vi "CfgFile Create Language File Chinese.vi"(8 "error in (no error)":errorcluster, 11 "LF2R IDE in":refnum<class "LF2R IDE.lvclass">) -> (0 "error out":errorcluster, 3 "LF2R IDE out":refnum<class "LF2R IDE.lvclass">)   [LabVIEW 2018, in "LF2R IDE.lvlib" / "LF2R IDE.lvclass"]
uses:
  LF2R IDE.lvclass
  0fceaff6-5102-487b-a0d8-62e3909835e7.vi
  <vilib>/JDP Science/JSONtext/Variant to JSON Text.vi
  <vilib>/JDP Science/JSONtext/LVClass Serializer/JSONtext LVClass Serializer.lvclass
  <vilib>/JDP Science/JSONtext/JSONtext.lvlib
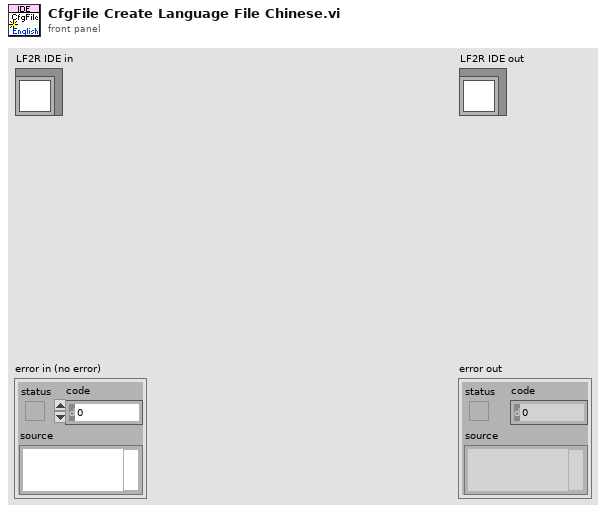
[diagram p1: front panel]
types:
  T1 = enum16{"open", "replace", "create", "open or create", "replace or create", "replace or create with confirmation"}
  T2 = typedef "LF2R IDE.lvlib/LF2R IDE.lvclass/Const UI Description Setting.ctl" = cluster{"Title":T3, "Frame Basic":T5, "Frame Skill":T6, "bp":T7, "w":T8, "b":T9, "i":T10, "o":T11, "c":T12, "Other":T13, "Menu":T14}
  T3 = typedef "LF2R IDE.lvlib/LF2R IDE.lvclass/Const UI Desc Frame Title.ctl" = cluster{"Frame Num":T4, "Name":T4}
  T4 = typedef "LF2R IDE.lvlib/LF2R IDE.lvclass/Const UI Desc Property.ctl" = cluster{"Name":string, "Tip":string, "Description":string}
  T5 = typedef "LF2R IDE.lvlib/LF2R IDE.lvclass/Const UI Desc Frame Basic.ctl" = cluster{"pic":T4, "state":T4, "wait":T4, "next":T4, "dvx":T4, "dvy":T4, "dvz":T4, "centerx":T4, "centery":T4, "sound":T4}
  T6 = typedef "LF2R IDE.lvlib/LF2R IDE.lvclass/Const UI Desc Frame Skill.ctl" = cluster{"mp":T4, "hit_a":T4, "hit_d":T4, "hit_j":T4, "hit_Fa":T4, "hit_Ua":T4, "hit_Da":T4, "hit_Fj":T4, "hit_Uj":T4, "hit_Dj":T4, "hit_ja":T4}
  T7 = typedef "LF2R IDE.lvlib/LF2R IDE.lvclass/Const UI Desc Frame bp.ctl" = cluster{"x":T4, "y":T4}
  T8 = typedef "LF2R IDE.lvlib/LF2R IDE.lvclass/Const UI Desc Frame w.ctl" = cluster{"kind":T4, "x":T4, "y":T4, "weaponact":T4, "cover":T4, "dvx":T4, "dvy":T4, "dvz":T4, "attacking":T4}
  T9 = typedef "LF2R IDE.lvlib/LF2R IDE.lvclass/Const UI Desc Frame b.ctl" = cluster{"kind":T4, "x":T4, "y":T4, "w":T4, "h":T4, "index":T4}
  T10 = typedef "LF2R IDE.lvlib/LF2R IDE.lvclass/Const UI Desc Frame i.ctl" = cluster{"kind":T4, "x":T4, "y":T4, "w":T4, "h":T4, "zwidth":T4, "dvx":T4, "dvy":T4, "dvz":T4, "fall":T4, "arest":T4, "vrest":T4, "bdefend":T4, "injury":T4, "effect":T4, "catchingact 1":T4, "catchingact 2":T4, "caughtact 1":T4, "caughtact 2":T4, "index":T4}
  T11 = typedef "LF2R IDE.lvlib/LF2R IDE.lvclass/Const UI Desc Frame o.ctl" = cluster{"kind":T4, "x":T4, "y":T4, "action":T4, "dvx":T4, "dvy":T4, "dvz":T4, "oid":T4, "facing":T4}
  T12 = typedef "LF2R IDE.lvlib/LF2R IDE.lvclass/Const UI Desc Frame c.ctl" = cluster{"kind":T4, "x":T4, "y":T4, "injury":T4, "cover":T4, "vaction":T4, "aaction":T4, "taction":T4, "hurtable":T4, "decrease":T4, "fronthurtact":T4, "backhurtact":T4, "throwvx":T4, "throwvy":T4, "throwvz":T4, "throwinjury":T4, "dircontrol":T4}
  T13 = typedef "LF2R IDE.lvlib/LF2R IDE.lvclass/Const UI Desc Other.ctl" = cluster{"File Path":T4, "GoTo":T4, "Apply Change":T4, "To Next Frame":T4}
  T14 = typedef "LF2R IDE.lvlib/LF2R IDE.lvclass/Const UI Desc Menu.ctl" = cluster{"File":T4, "Open File":T4, "Save File":T4, "Exit":T4, "Settings":T4, "Preferences":T4, "Help":T4, "Show Context Help":T4}
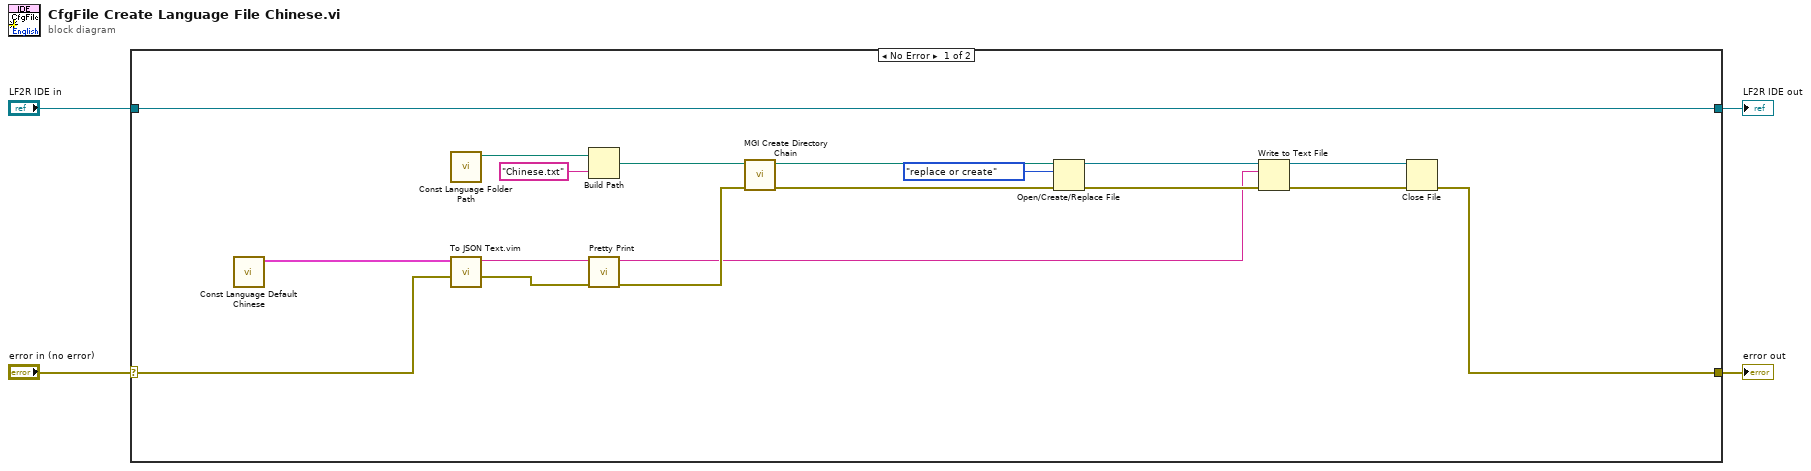
[diagram p0: block diagram]
diagram:
  n1 = case shown="No Error" "error in (no error)" {
    selector: "error in (no error)" -> [w18 w24]
    tunnel: [w9 w24] -> w3
    tunnel: [w22 w23] -> w1
    tunnel: "LF2R IDE in" -> [w22 w23]
    frame No Error {
      n2 = call "Const Language Default Chinese.vi"() -> ("UI Descriptions"=w5:T2)  [unwired: 11 in]
      n3 = call "Const Language Folder Path.vi"() -> ("Language Folder Path"=w8:path)  [unwired: 11 in]
      n4 = call "To JSON Text.vim"("error in (no error)"=w18, "Anything"=w5) -> ("error out"=w20:errorcluster, "<JSON>"=w21:string)  [unwired: 8 in]
      n5 = Build Path(base path=w8, name or relative path="Chinese.txt") -> (appended path=w6:path)
      n6 = call <vilib>:"Pretty Print.vi"("error in (no error)"=w20, "JSON"=w21) -> ("error out"=w19:errorcluster, "<JSON>"=w10:string)  [unwired: 7 in, 1 out]
      n7 = call <userlib>:"MGI Create Directory Chain.vi"("Error In"=w19, "Path"=w6) -> ("Error Out"=w11:errorcluster, "Duplicate Path"=w12:path)  [unwired: 8 in]
      n8 = Open/Create/Replace File(file path (use dialog)=w12, error in=w11, operation (0:open)=T1."replace or create") -> (refnum out=w17:refnum<file>, error out=w16:errorcluster)  [unwired: 3 in, 1 out]
      n9 = Write to Text File(file (use dialog)=w17, text=w10, error in=w16) -> (refnum out=w15:refnum<file>, error out=w14:errorcluster)  [unwired: 1 in, 1 out]
      n10 = Close File(refnum=w15, error in=w14) -> (error out=w9:errorcluster)  [unwired: 1 out]
    }
    frame Error {
    }
  }
  "error out" <- w3
  "LF2R IDE out" <- w1
